vi "16CH Data Array.vi"(10 "Relays 9-16":bool[](array[boolean]), 11 "Relays 1-8":bool[](array[boolean])) -> (1 "Relays 1-16":bool[](array[boolean]), 3 "unsigned byte array":u8[](array[numeric]))   [LabVIEW 2020]
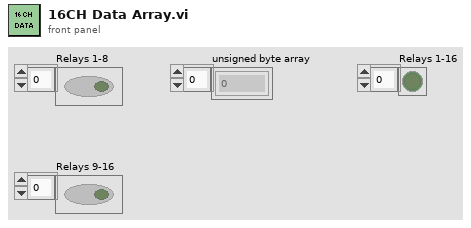
[diagram p1: front panel]
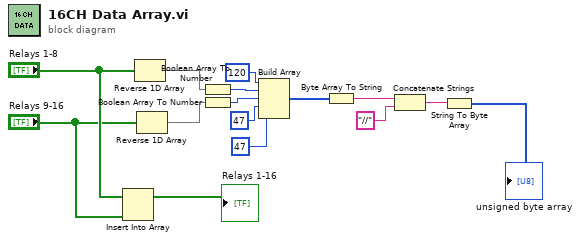
[diagram p0: block diagram]
diagram:
  n1 = Insert Into Array(array="Relays 1-8", new element="Relays 9-16") -> (→"Relays 1-16":bool[])  [unwired: 1 in]
  n2 = Reverse 1D Array(array="Relays 1-8") -> (reversed array=w5:bool[])
  n3 = Reverse 1D Array(array="Relays 9-16") -> (reversed array=w4:bool[])
  n4 = Boolean Array To Number(Boolean array=w5) -> (number=w6:u32)
  n5 = Boolean Array To Number(Boolean array=w4) -> (number=w15:u32)
  n6 = Build Array(u32 120 ("element"), w6, w15, u32 47 ("element"), u32 47 ("element")) -> (w10:u32[])
  n7 = Byte Array To String(unsigned byte array=w10) -> (string=w11:string)
  n8 = Concatenate Strings(w11, "//" ("string")) -> (w13:string)
  n9 = String To Byte Array(string=w13) -> (unsigned byte array=→"unsigned byte array":u8[])
